vi "Write Account Number.vi"(8 "error in (no error)":errorcluster, 10 "Account Number":string, 11 "SQS in":refnum<class "NI_AWS_SQS.lvclass">) -> (0 "error out":errorcluster, 3 "SQS out":refnum<class "NI_AWS_SQS.lvclass">)   [LabVIEW 2015, in "NI_AWS_SQS.lvclass"]
uses:
  NI_AWS_SQS.lvclass
  NI_AWS_SQS.lvclass/NI_AWS_SQS.ctl
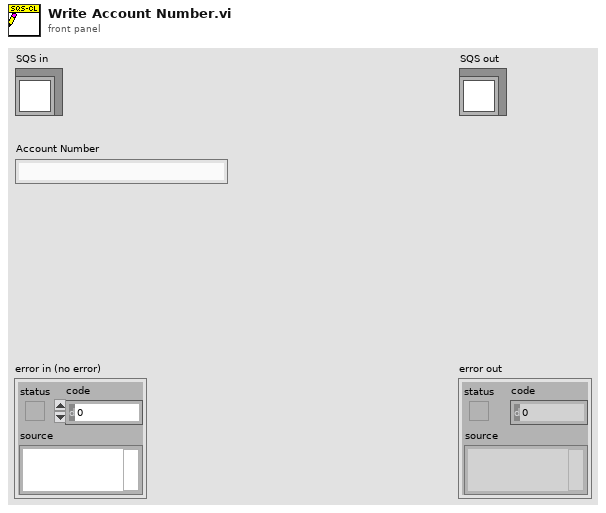
[diagram p1: front panel]
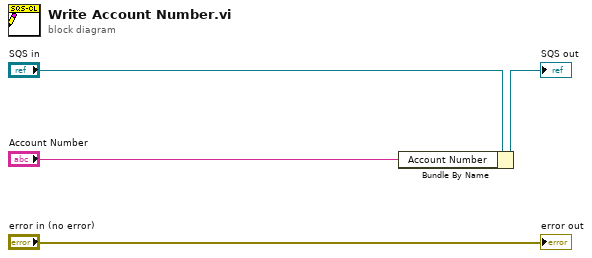
[diagram p0: block diagram]
diagram:
  n1 = Bundle By Name(cluster="SQS in", "Account Number"="Account Number") -> (→"SQS out":refnum<class "NI_AWS_SQS.lvclass">)
  "error out" <- "error in (no error)"
